vi "Verify Status.vi"(8 "Error In":errorcluster, 9 "States":T2(ring), 10 "GEA Inputs":T1={"Source"=228, "Destination"=36} {"Destination" format="%.0x"; "Source" format="%.0x"}, 11 "GEA2 Reference In":refnum<k24>) -> (0 "Error Out":errorcluster, 1 "Pass/Fail":bool, 2 "Report Text":string, 3 "GEA2 Reference Out":refnum<k24>)   [LabVIEW 2016]
uses:
  Common/LabVIEW GEA2 Toolkit/LabVIEW_GEA2_Toolkit.lvlibp/type defs/Source_Destination.ctl
  Q:/Common/DLLs/GEA3/GeaCommunication.dll
  Common/DLLs/GEA3/GeaCommunication.dll
  Common/LabVIEW GEA2 Toolkit/LabVIEW_GEA2_Toolkit.lvlibp/type defs/ERD Read Data In.ctl
  Common/LabVIEW GEA2 Toolkit/LabVIEW_GEA2_Toolkit.lvlibp/type defs/Data Type.ctl
  Common/LabVIEW GEA2 Toolkit/LabVIEW_GEA2_Toolkit.lvlibp
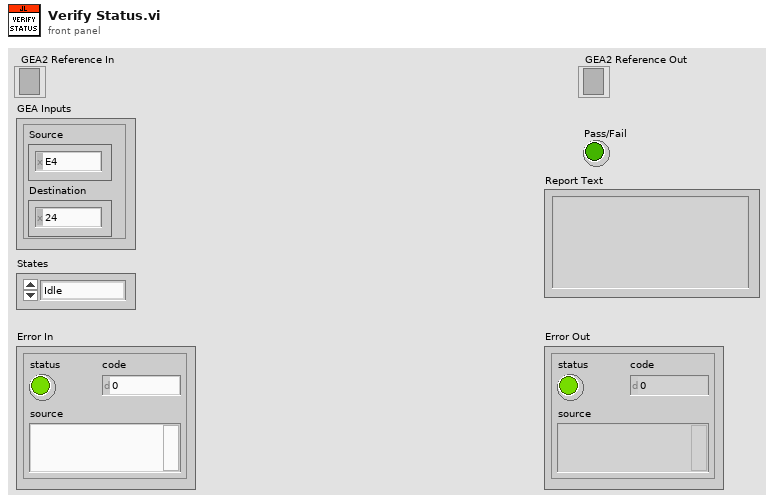
[diagram p1: front panel]
types:
  T1 = typedef "LabVIEW_GEA2_Toolkit.lvlibp/Source_Destination.ctl" = cluster{"Source":u8, "Destination":u8}
  T2 = enum16{"Idle", "Standby", "Run", "Pause", "EOC", "DSM_DelayRun", "DelayRun", "DelayPause", "DrainTimeout", "CleanSpeak"}
  T3 = typedef "LabVIEW_GEA2_Toolkit.lvlibp/ERD Read Data In.ctl" = cluster{"ERD Number":u16, "Data Type":T4}
  T4 = typedef "LabVIEW_GEA2_Toolkit.lvlibp/Data Type.ctl" = enum16{"string", "boolean", "uint8_t", "uint16_t", "uint32_t", "uint64_t", "int8_t", "int16_t", "int32_t", "int64_t"}
  T5 = typedef "LabVIEW_GEA2_Toolkit.lvlibp/ERD Read Data Out.ctl" = cluster{"ERD Number":u16, "Data":string}
  T6 = cluster{"ERD Data Out[0]":T5, "ERD Data Out[1]":T5, "ERD Data Out[2]":T5, "ERD Data Out[3]":T5, "ERD Data Out[4]":T5, "ERD Data Out[5]":T5, "ERD Data Out[6]":T5, "ERD Data Out[7]":T5, "ERD Data Out[8]":T5}
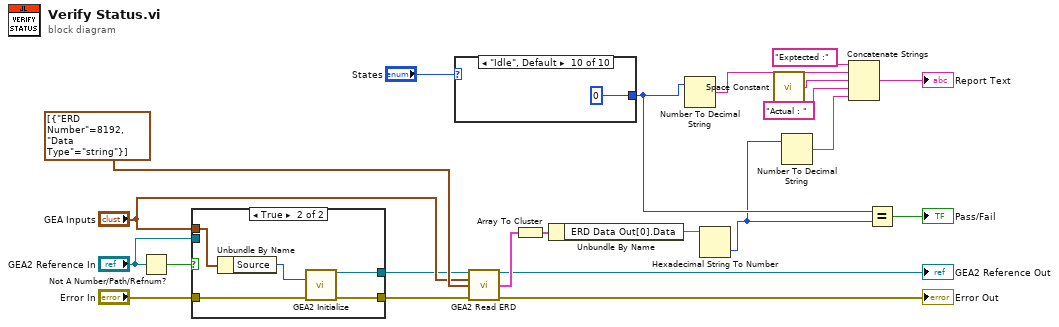
[diagram p0: block diagram]
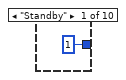
[diagram p3: hidden frame]
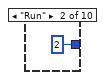
[diagram p4: hidden frame]
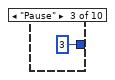
[diagram p5: hidden frame]
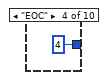
[diagram p6: hidden frame]
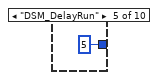
[diagram p7: hidden frame]
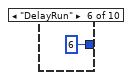
[diagram p8: hidden frame]
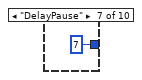
[diagram p9: hidden frame]
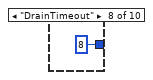
[diagram p10: hidden frame]
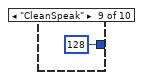
[diagram p11: hidden frame]
diagram:
  n1 = Not A Number/Path/Refnum?(number/path/refnum="GEA2 Reference In") -> (NaN/Path/Refnum?=w18:bool)
  n2 = case shown="True" w18 {
    tunnel: "Error In" -> [w23 w29]
    tunnel: [w23 w28] -> w12
    tunnel: "GEA2 Reference In" -> [w24 _]
    tunnel: [w24 w27] -> w13
    tunnel: "GEA Inputs" -> [_ w26]
    frame False {
    }
    frame True {
      n3 = Unbundle By Name(w26) -> ("Source"=w25:u8)
      n4 = call "GEA2 Initialize.vi"("Source Address"=w25, "error in"=w29) -> ("GEA2 Reference Out"=w27:refnum<k24>, "error out"=w28:errorcluster)  [unwired: 11 in, 1 out]
    }
  }
  n5 = case shown="\"Idle\", Default" "States" {
    tunnel: [u8 1 u8 2 u8 3 u8 4 u8 5 u8 6 u8 7 u8 8 u8 128 u8 0] -> w9
    frame "Standby" {
    }
    frame "Run" {
    }
    frame "Pause" {
    }
    frame "EOC" {
    }
    frame "DSM_DelayRun" {
    }
    frame "DelayRun" {
    }
    frame "DelayPause" {
    }
    frame "DrainTimeout" {
    }
    frame "CleanSpeak" {
    }
    frame "Idle", Default {
    }
  }
  n6 = call "GEA2 Read ERD.vi"("GEA2 Reference In"=w13, "GEA Inputs"="GEA Inputs", "Read ERD List"=T3[] [{"ERD Number"=8192, "Data Type"=enum."string"}], "Error In"=w12) -> ("GEA2 Reference Out"=→"GEA2 Reference Out":refnum<k24>, "ERD Data Out"=w21:T5[], "Error Out"=→"Error Out":errorcluster)  [unwired: 8 in, 1 out]
  n7 = Array To Cluster(array=w21) -> (cluster=w20:T6)
  n8 = Unbundle By Name(w20) -> ("ERD Data Out[0].Data"=w5:string)
  n9 = Number To Decimal String(number=w9) -> (decimal integer string=w8:string)  [unwired: 1 in]
  n10 = Hexadecimal String To Number(string=w5) -> (number=w2:u32)  [unwired: 2 in, 1 out]
  n11 = call <vilib>:"Space Constant.vi"() -> ("String"=w7:string)
  n12 = Number To Decimal String(number=w2) -> (decimal integer string=w1:string)  [unwired: 1 in]
  n13 = Concatenate Strings("Exptected :", w8, w7, "Actual : ", w1) -> (→"Report Text":string)
  n14 = Equal?(x=w9, y=w2) -> (x = y?=→"Pass/Fail":bool)
